vi "RemoveInstance.vi"(7 "Logger Name (Logger)":string="Logger", 8 "error in (no error)":errorcluster) -> (0 "error out":errorcluster, 3 "RQMHLogger Get":refnum<class "Logger.lvclass">)   [LabVIEW 2024, in "LogSingleton.lvlib"]
uses:
  LogSingleton.lvlib
  RQMHLogger/Logger.lvclass
  fgvCommands.ctl
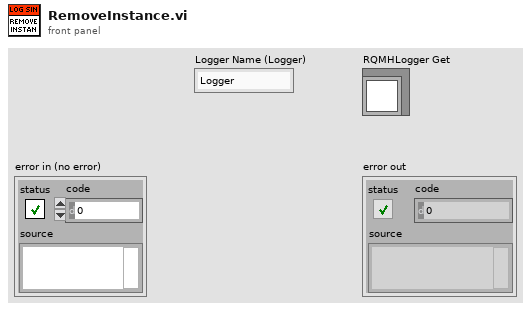
[diagram p1: front panel]
types:
  T1 = typedef "LogSingleton.lvlib/fgvCommands.ctl" = enum16{"Add", "Get", "GetAllKeys", "Remove"}
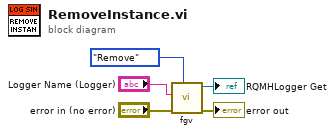
[diagram p0: block diagram]
diagram:
  n1 = call "fgv.vi"("fgv command"=fgvCommands."Remove", "error in (no error)"="error in (no error)", "Logger Name"="Logger Name (Logger)") -> ("error out"=→"error out":errorcluster, "RQMHLogger Get"=→"RQMHLogger Get":refnum<class "Logger.lvclass">)  [unwired: 6 in, 1 out]
